vi "Current Value.vi"(8 "error in (no error)":errorcluster, 11 "Channel in":refnum<class "Channel.lvclass">) -> (0 "error out":errorcluster, 2 "Value":T1 {"Timestamp" format="%<%H:%M:%S%3u>T"}, 3 "Channel out":refnum<class "Channel.lvclass">)   [LabVIEW 2020, in "Vecto.lvlib" / "Channel.lvclass"]
uses:
  Channel.lvclass
  Channel Value.ctl
  Channel.lvclass/Channel.ctl
  Vecto.lvlib
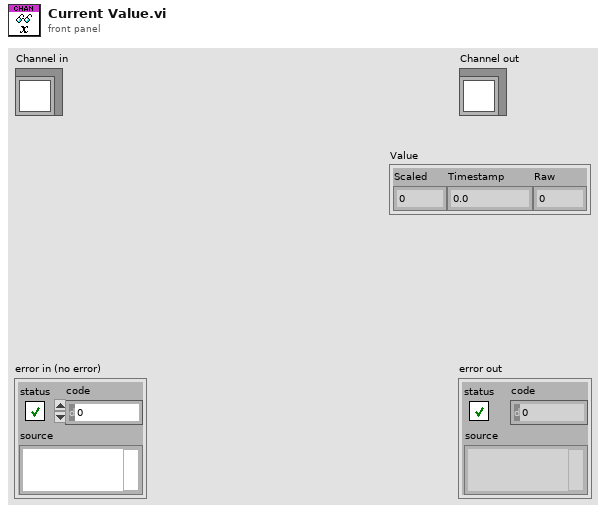
[diagram p1: front panel]
types:
  T1 = typedef "Vecto.lvlib/Channel Value.ctl" = cluster{"Scaled":dbl, "Timestamp":dbl, "Raw":dbl}
  T2 = typedef "Vecto.lvlib/Channel.ctl" = cluster{"Info":T3, "Value":T1}
  T3 = typedef "Vecto.lvlib/Channel Info.ctl" = cluster{"Name":string, "Group":string, "Owning Node":u32, "Owning Task":u32, "Resource":string}
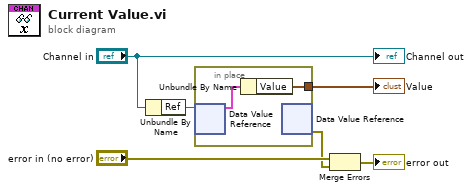
[diagram p0: block diagram]
diagram:
  n1 = Unbundle By Name("Channel in") -> ("Ref"=w4:refnum<data-value>)
  n2 = in-place {
    in-place-border: [w7] -> w1
    n3 = in-place-dvr #1(w4) -> (w8:T2)  [unwired: 1 out]
    n4 = Unbundle By Name(w8) -> ("Value"=w7:T1)
    n5 = in-place-dvr #1() -> (w2:errorcluster)  [unwired: 1 in, 1 out]
  }
  "Value" <- w1
  n6 = Merge Errors("error in (no error)", w2) -> (→"error out":errorcluster)
  "Channel out" <- "Channel in"
